vi "OOP Server Example.vi"() -> ()   [LabVIEW 2019, in "OOP Server.lvlib"]
uses:
  OOP Server.lvlib
  Class/OOP Server.lvclass/OOP Server.ctl
  Class/OOP Server.lvclass
panel:
  in  "Enable Async Mode":bool
  out "error out":errorcluster
  in  "Stop":bool
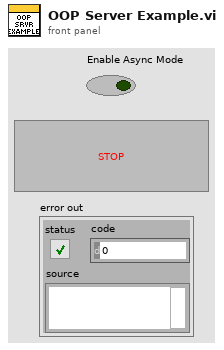
[diagram p1: front panel]
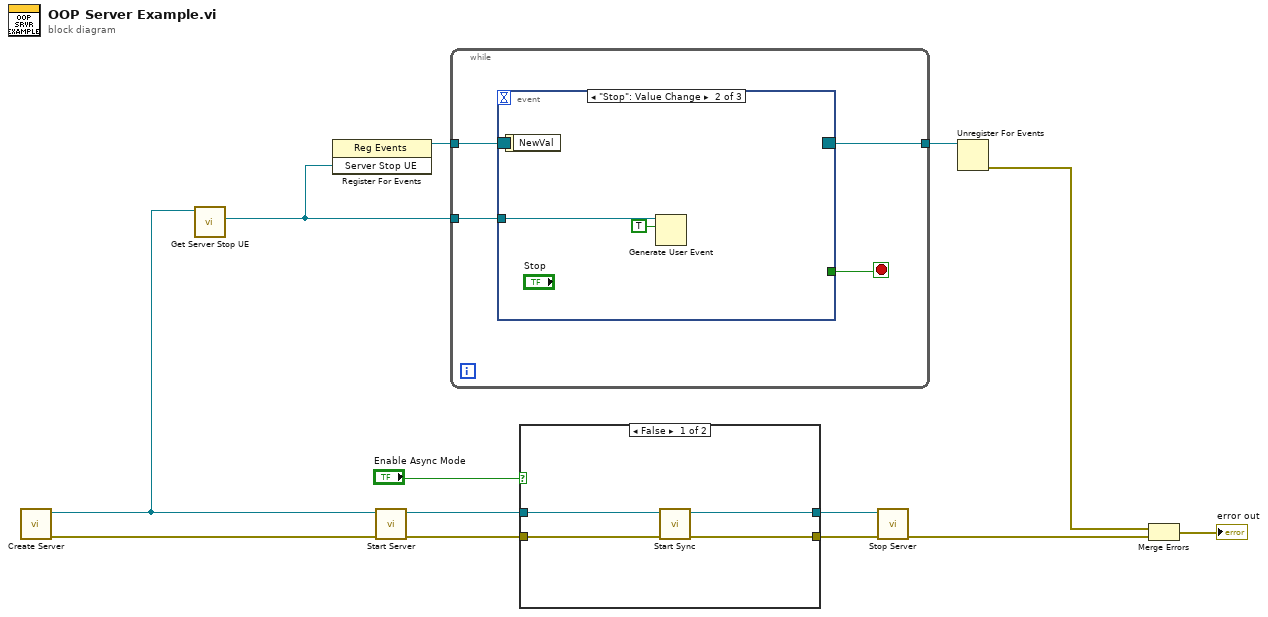
[diagram p0: block diagram]
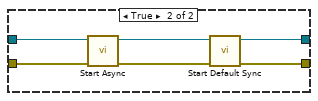
[diagram p2: hidden frame]
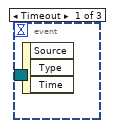
[diagram p3: hidden frame]
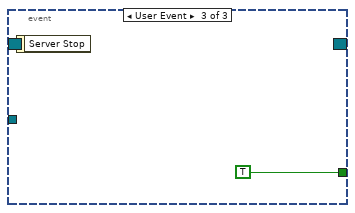
[diagram p4: hidden frame]
diagram:
  n1 = call "Create Server.vi"() -> ("error out"=w1:errorcluster, "OOP Server out"=w2:refnum<class "OOP Server.lvclass">)  [unwired: 10 in]
  n2 = call "Get Server Stop UE.vi"("OOP Server in"=w2) -> ("Server Stop UE"=w10:refnum<user-event>)  [unwired: 9 in, 1 out]
  n3 = register-events(w10) -> (reference out=w11:refnum<event-registration>)  [unwired: 2 in, 1 out]
  n4 = call "Start Server.vi"("error in (no error)"=w1, "OOP Server in"=w2) -> ("error out"=w5:errorcluster, "OOP Server out"=w4:refnum<class "OOP Server.lvclass">)  [unwired: 8 in]
  n5 = while {
    tunnel: w10 -> [w17]
    tunnel: w11 -> [w16]
    tunnel: [w14] -> w9
    stop <- w15 stop-if-true
    n6 = event shown="[1] \"Stop\": Value Change" {
      selector: w16 -> [_ _ _]
      dyn-events: [_ _ _] -> w14
      timeout: _ -> [_ _ _]
      tunnel: w17 -> [_ w19 _]
      tunnel: [_ _ TRUE] -> w15
      event Timeout {
        n7 = event-data() -> ()  [unwired: 1 in, 3 out]
      }
      event "Stop": Value Change {
        n8 = event-data() -> ()  [unwired: 1 in, 1 out]
        n9 = Generate User Event(user event=w19, event data cluster=TRUE ("event data")) -> ()  [unwired: 2 in, 2 out]
      }
      event User Event {
        n10 = event-data() -> ()  [unwired: 1 in, 1 out]
      }
    }
  }
  n11 = case shown="False" "Enable Async Mode" {
    tunnel: [w21 w30] -> w13
    tunnel: [w22 w29] -> w12
    tunnel: w5 -> [w24 w28]
    tunnel: w4 -> [w23 w27]
    frame False {
      n12 = call "Start Sync.vi"("error in (no error)"=w24, "OOP Server in"=w23) -> ("error out"=w21:errorcluster, "OOP Server out"=w22:refnum<class "OOP Server.lvclass">)  [unwired: 8 in]
    }
    frame True {
      n13 = call "Start Async.vi"("error in (no error)"=w28, "OOP Server in"=w27) -> ("error out"=w26:errorcluster, "OOP Server out"=w25:refnum<class "OOP Server.lvclass">)  [unwired: 8 in]
      n14 = call "Start Default Sync.vi"("error in (no error)"=w26, "OOP Server in"=w25) -> ("error out"=w30:errorcluster, "OOP Server out"=w29:refnum<class "OOP Server.lvclass">)  [unwired: 8 in]
    }
  }
  n15 = call "Stop Server.vi"("error in (no error)"=w13, "OOP Server in"=w12) -> ("error out"=w8:errorcluster)  [unwired: 8 in, 1 out]
  n16 = Unregister For Events(event registration refnum=w9) -> (error out=w7:errorcluster)  [unwired: 1 in]
  n17 = Merge Errors(w7, w8) -> (→"error out":errorcluster)
